vi "Periodic Tasks.vi"(8 "error in":errorcluster) -> ()   [LabVIEW 2015]
doc: "This VI runs in parallel to other tasks. It can contain as many user-defined periodic loops as you need. These can carry out PID or other sorts of timed response."
uses:
  <vilib>/Rock Robotics/WPI/Utilities/WPI_GetSetVariantRefNum.vi
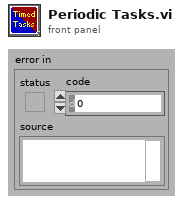
[diagram p1: front panel]
types:
  T1 = typedef "WPI_MotorControlDeviceRef.ctl" = cluster{"DeviceStatus":errorcluster, "Type":T2, "PWM":cluster{"PWM Channel":T3, "DeadBand":T4}, "CAN":cluster{"Device Number":u8, "Control Mode":T5, "Semaphore":T6, "Max Vout":dbl, "TalonSRX Control Mode":T7}, "Invert":bool}
  T2 = typedef "WPI_MotorControlType.ctl" = enum16{"PWM", "CAN", "CANTalonSRX"}
  T3 = typedef "FPGA_DIOPWMChannel.ctl" = enum8{"PWM 0", "PWM 1", "PWM 2", "PWM 3", "PWM 4", "PWM 5", "PWM 6", "PWM 7", "PWM 8", "PWM 9", "PWM MXP 0", "PWM MXP 1", "PWM MXP 2", "PWM MXP 3", "PWM MXP 4", "PWM MXP 5", "PWM MXP 6", "PWM MXP 7", "PWM MXP 8", "PWM MXP 9", "Invalid"}
  T4 = typedef "WPI_PWMDeadband.ctl" = cluster{"Name":string, "maxPositivePwm":i32, "minPositivePwm":i32, "centerPwm":i32, "maxNegativePwm":i32, "minNegativePwm":i32, "angularRange":u16}
  T5 = typedef "WPI_CANJaguar_ControlMode.ctl" = enum8{"Percent VBus", "Current", "Speed", "Position", "Voltage"}
  T6 = typedef "Semaphore RefNum" = refnum<k1>
  T7 = typedef "WPI_CANTalonSRX_APIControlMode.ctl" = enum8{"Percent VBus", "Speed", "Position", "Slave", "Unchanged / Invalid", "Voltage Compensation", "Current", "Motion Profile"}
  T8 = typedef "WPI_AccelerometerDevRef.ctl" = cluster{"DevStatus":errorcluster, "Scaling":T9, "Analog Channels":T10, "I2C Bus":T12, "SPI Bus":T13, "Accel Range":T14, "ADXL Axes":T15, "Handle":i32, "Device Address":u8, "Accel Type":enum16{"Analog", "ADXL345 I2C", "ADXL345 SPI", "Internal", "ADXL362 SPI"}}
  T9 = typedef "WPI_AccelerometerScaling.ctl" = cluster{"Gain (VoltsPerG)":dbl, "Center Voltage":dbl}
  T10 = typedef "WPI_AccelerometerAnalogChannels.ctl" = cluster{"X-Axis":T11, "Y-Axis":T11, "Z-Axis":T11}
  T11 = typedef "FPGA_AIChannel.ctl" = enum8{"AI 0", "AI 1", "AI 2", "AI 3", "AI MXP 0", "AI MXP 1", "AI MXP 2", "AI MXP 3", "Invalid"}
  T12 = typedef "i2c_bus.ctl" = enum16{"I2C On-Board", "I2C MXP", "Invalid"}
  T13 = typedef "spi_bus.ctl" = enum16{"SPI On-Board, CS0", "SPI On-Board, CS1", "SPI On-Board, CS2", "SPI On-Board, CS3", "SPI MXP", "Invalid"}
  T14 = typedef "ADXL345 Range.ctl" = u8
  T15 = typedef "WPI_AccelerometerADXL345 Axes.ctl" = cluster{"X-Axis":bool, "Y-Axis":bool, "Z-Axis":bool}
  T16 = typedef "WPI_JoystickDevRef.ctl" = cluster{"Device":T17}
  T17 = typedef "WPI_JoystickDeviceEnum.ctl" = enum16{"USB 0", "USB 1", "USB 2", "USB 3", "USB 4", "USB 5"}
  T18 = cluster{"AccelerometerDevRef":T8, "JoystickDevRef":T16, "JoystickDevRef":T16, "MotorControlDevRef":T1, "MotorControlDevRef":T1, "MotorControlDevRef":T1, "MotorControlDevRef":T1, "MotorControlDevRef":T1, "MotorControlDevRef":T1, "MotorControlDevRef":T1, "MotorControlDevRef":T1, "MotorControlDevRef":T1, "MotorControlDevRef":T1}
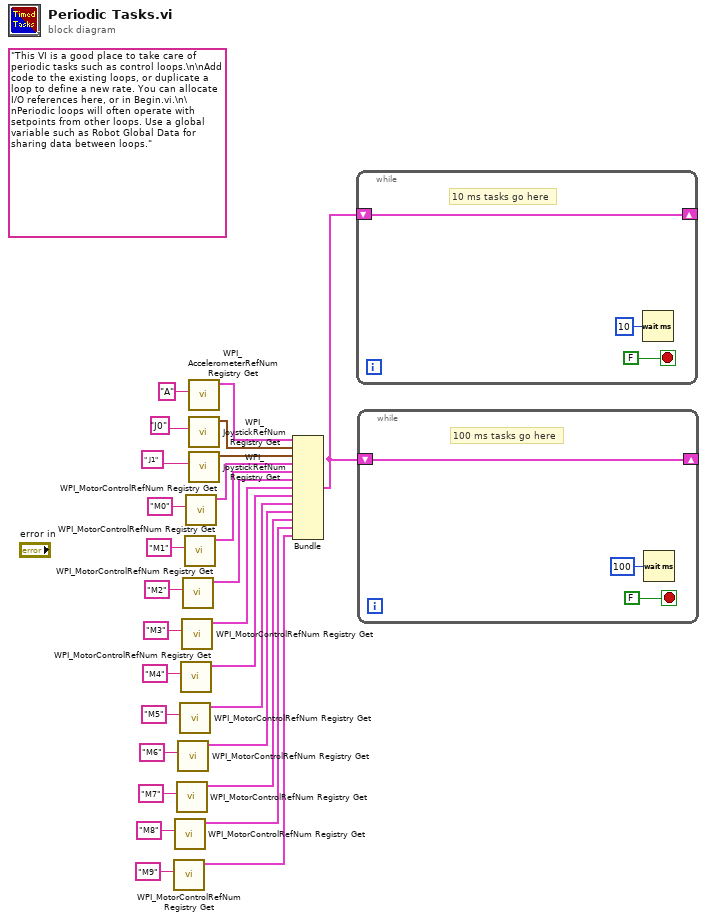
[diagram p0: block diagram]
diagram:
  (unwired) "This VI is a good place to take care of periodic tasks such as control loops.\n\nAdd code to the existing loops, or duplicate a loop to define a new rate. You can allocate I/O references here, or in Begin.vi.\n\nPeriodic loops will often operate with setpoints from other loops. Use a global variable such as Robot Global Data for sharing data between loops."
  n1 = call <vilib>:"WPI_MotorControlRefNum Registry Get.vi"("refnum name"="M9") -> ("MotorControlDevRef"=w3:T1)  [unwired: 9 in, 1 out]
  n2 = call <vilib>:"WPI_MotorControlRefNum Registry Get.vi"("refnum name"="M8") -> ("MotorControlDevRef"=w4:T1)  [unwired: 9 in, 1 out]
  n3 = call <vilib>:"WPI_MotorControlRefNum Registry Get.vi"("refnum name"="M7") -> ("MotorControlDevRef"=w7:T1)  [unwired: 9 in, 1 out]
  n4 = call <vilib>:"WPI_MotorControlRefNum Registry Get.vi"("refnum name"="M6") -> ("MotorControlDevRef"=w8:T1)  [unwired: 9 in, 1 out]
  n5 = call <vilib>:"WPI_MotorControlRefNum Registry Get.vi"("refnum name"="M5") -> ("MotorControlDevRef"=w11:T1)  [unwired: 9 in, 1 out]
  n6 = call <vilib>:"WPI_MotorControlRefNum Registry Get.vi"("refnum name"="M4") -> ("MotorControlDevRef"=w12:T1)  [unwired: 9 in, 1 out]
  n7 = call <vilib>:"WPI_MotorControlRefNum Registry Get.vi"("refnum name"="M3") -> ("MotorControlDevRef"=w13:T1)  [unwired: 9 in, 1 out]
  n8 = call <vilib>:"WPI_MotorControlRefNum Registry Get.vi"("refnum name"="M2") -> ("MotorControlDevRef"=w14:T1)  [unwired: 9 in, 1 out]
  n9 = call <vilib>:"WPI_MotorControlRefNum Registry Get.vi"("refnum name"="M1") -> ("MotorControlDevRef"=w23:T1)  [unwired: 9 in, 1 out]
  n10 = call <vilib>:"WPI_MotorControlRefNum Registry Get.vi"("refnum name"="M0") -> ("MotorControlDevRef"=w19:T1)  [unwired: 9 in, 1 out]
  n11 = call <vilib>:"WPI_AccelerometerRefNum Registry Get.vi"("refnum name"="A") -> ("AccelerometerDevRef"=w1:T8)  [unwired: 9 in, 1 out]
  n12 = call <vilib>:"WPI_JoystickRefNum Registry Get.vi"("refnum name"="J0") -> ("JoystickDevRef"=w21:T16)  [unwired: 1 in, 9 out]
  n13 = call <vilib>:"WPI_JoystickRefNum Registry Get.vi"("refnum name"=" J1") -> ("JoystickDevRef"=w26:T16)  [unwired: 1 in, 9 out]
  n14 = Bundle("AccelerometerDevRef"=w1, "JoystickDevRef"=w21, "JoystickDevRef"=w26, "MotorControlDevRef"=w19, "MotorControlDevRef"=w23, "MotorControlDevRef"=w14, "MotorControlDevRef"=w13, "MotorControlDevRef"=w12, "MotorControlDevRef"=w11, "MotorControlDevRef"=w8, "MotorControlDevRef"=w7, "MotorControlDevRef"=w4, "MotorControlDevRef"=w3) -> (w25:T18)  [unwired: 1 out]
  n15 = while {
    shift-right: [w28] -> _
    shift-left: w25 -> [w28]
    stop <- FALSE stop-if-true
    # "10 ms tasks go here"
    n16 = Wait (ms)(milliseconds to wait=u32 10) -> ()  [unwired: 1 out]
  }
  n17 = while {
    shift-right: [w31] -> _
    shift-left: w25 -> [w31]
    stop <- FALSE stop-if-true
    # "100 ms tasks go here"
    n18 = Wait (ms)(milliseconds to wait=u32 100) -> ()  [unwired: 1 out]
  }
